vi "Run API.vi"(8 "Error In":errorcluster, 11 "DVR Ref":T1[](array[typedef])) -> (0 "Error Out":errorcluster)   [LabVIEW 2023, in "Arithemetic Operation.lvclass"]
doc: "The VI acts as a wrapper to run all the UI VIs of different operations in the background."
uses:
  Arithemetic Operation.lvclass
  Typedef/DVR Ref.ctl
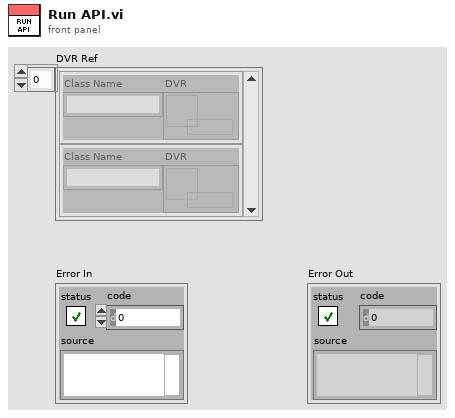
[diagram p1: front panel]
types:
  T1 = typedef "DVR Ref.ctl" = cluster{"Class Name":string, "DVR":refnum<data-value>}
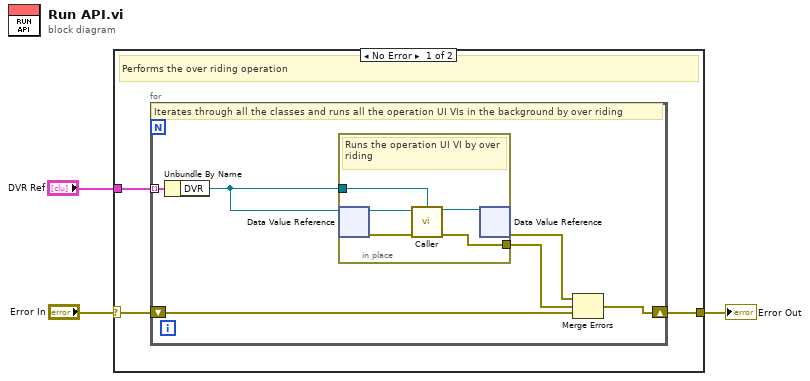
[diagram p0: block diagram]
diagram:
  n1 = case shown="No Error" "Error In" {
    selector: "Error In" -> [w6 w18]
    tunnel: [w5 w18] -> w2
    tunnel: "DVR Ref" -> [w4 _]
    frame No Error {
      # "Performs the over riding operation"
      n2 = for {
        tunnel: w4 -> [w12] mode=indexing
        shift-right: [w7] -> w5
        shift-left: w6 -> [w10]
        # "Iterates through all the classes and runs all the operation UI VIs in the background by over riding"
        n3 = Unbundle By Name(w12) -> ("DVR"=w11:refnum<data-value>)
        n4 = in-place {
          in-place-border: [w16] -> w9
          in-place-border: w11 -> [w13]
          # "Runs the operation UI VI by over riding"
          n5 = in-place-dvr #1(w11) -> (w15:refnum<class "Arithemetic Operation.lvclass">, w17:errorcluster)
          n6 = call-dynamic "Caller.vi"("Arithemetic Operation in"=w15, "DVR"=w13, "Error In"=w17) -> ("Arithemetic Operation out"=w14:refnum<class "Arithemetic Operation.lvclass">, "Error Out"=w16:errorcluster)  [unwired: 11 in]
          n7 = in-place-dvr #1(w14) -> (w8:errorcluster)  [unwired: 1 out]
        }
        n8 = Merge Errors(w8, w9, w10) -> (w7:errorcluster)
      }
    }
    frame Error {
    }
  }
  "Error Out" <- w2
